vi "proto1.vi"() -> ()   [LabVIEW 2020]
panel:
  out "PPG Monitor":cluster{dbl[], dbl[]}[](graph)
  out "Physiological Vitals":cluster{"heartrate":dbl, "SpO2":dbl}(graph)
  in  "Numer of Samples":i32(slide)=1000 min=1000 max=60002 step=100 scale=0.0..20000.0
  in  "PPG Dataset File Path":path
  out "SpO2 (%)":dbl
  out "Heart Rate (BPM)":dbl
  out "Time Period (seconds)":dbl
  in  "Influence":dbl=0.8
  in  "Lag":dbl=30.0
  in  "Threshold":dbl=3.4
  # "Physiological Vitals"
  # "Peak Detection Parameter"
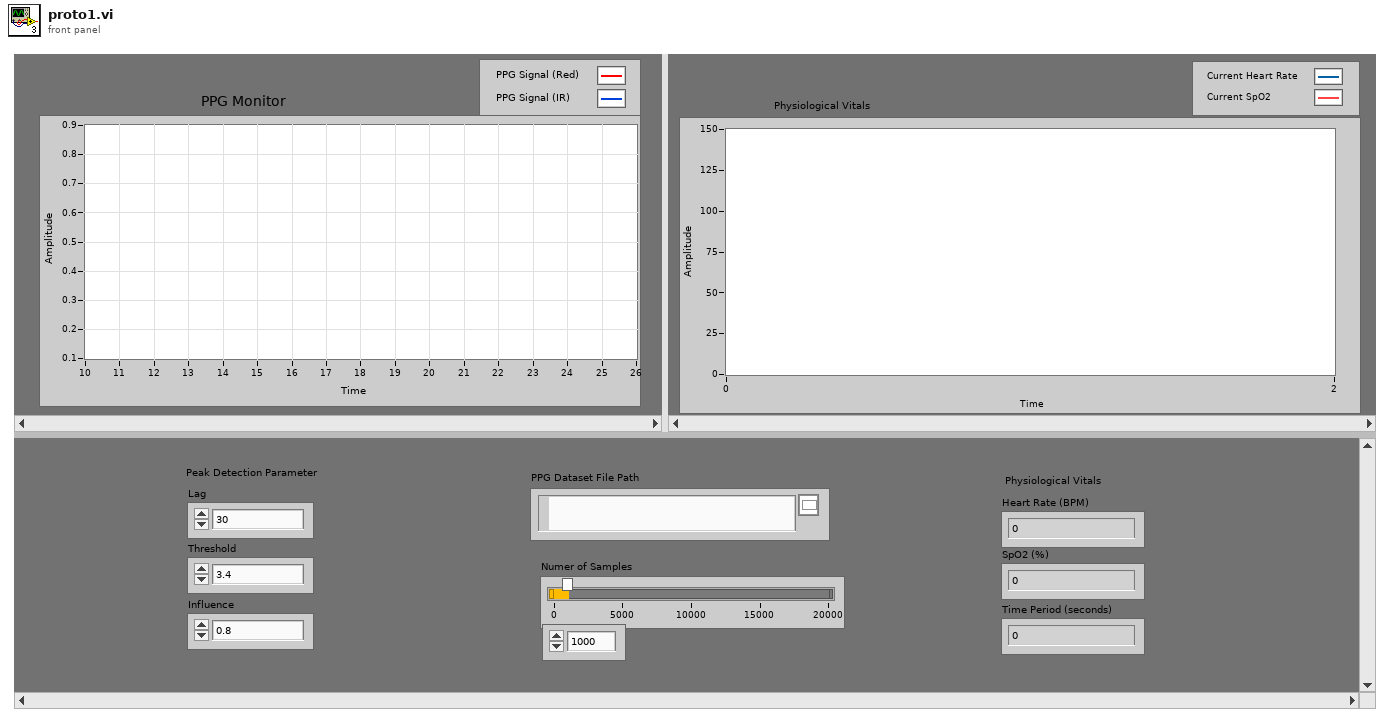
[diagram p1: front panel]
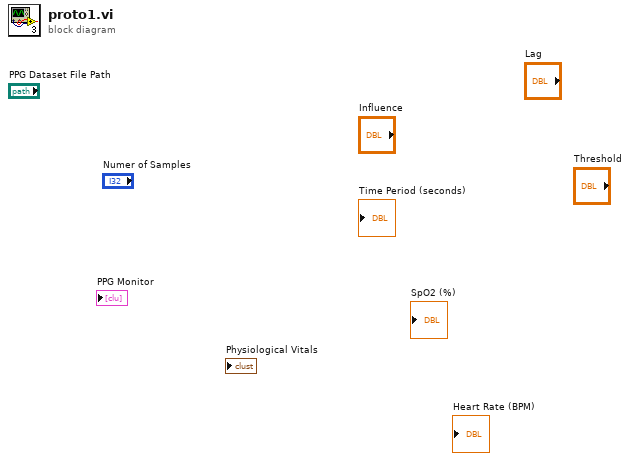
[diagram p0: block diagram]
diagram:
